vi "Calibration Mode.vi"(8 "error in (no error)":errorcluster, 10 "Enable":bool, 11 "ENET in":refnum<class "ENET_BS120x.lvclass">) -> (0 "error out":errorcluster, 3 "ENET out":refnum<class "ENET_BS120x.lvclass">)   [LabVIEW 2021, in "BS120x Driver.lvlib" / "ENET_BS120x.lvclass"]
doc: "Calibration mode disables the current calibration, removes all scaling, and returns bit counts."
uses:
  ENET_BS120x.lvclass
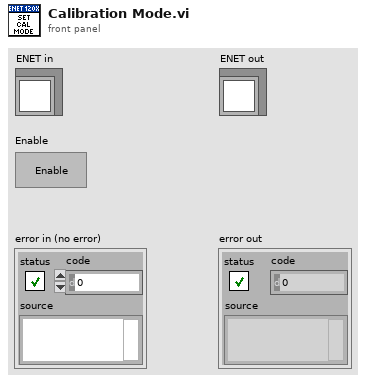
[diagram p1: front panel]
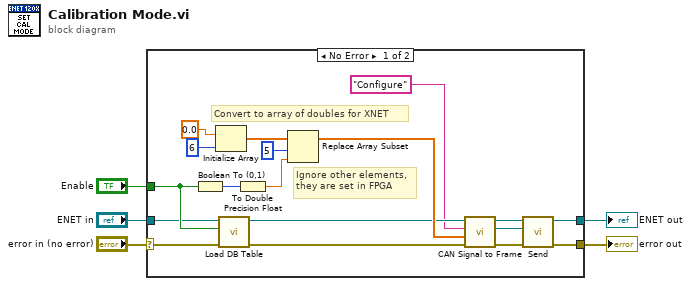
[diagram p0: block diagram]
diagram:
  n1 = case shown="No Error" "error in (no error)" {
    selector: "error in (no error)" -> [w23 w25]
    tunnel: [w8 w25] -> w4
    tunnel: [w9 w24] -> w2
    tunnel: "ENET in" -> [w15 w24]
    tunnel: "Enable" -> [w16 _]
    frame No Error {
      # "Ignore other elements,\nthey are set in FPGA"
      # "Convert to array of doubles for XNET"
      n2 = Boolean To (0,1)(Boolean=w16) -> (0, 1=w17:i16)
      n3 = Initialize Array(0.0 ("element"), 6 ("dimension size")) -> (w21:dbl[])
      n4 = call-dynamic "Load DB Table.vi"("error in (no error)"=w23, "Calibration Mode"=w16, "ENET in"=w15) -> ("error out"=w6:errorcluster, "ENET out"=w13:refnum<class "ENET_BS120x.lvclass">)  [unwired: 7 in]
      n5 = To Double Precision Float(number=w17) -> (double precision float=w22:dbl)
      n6 = Replace Array Subset(array=w21, new element=w22, index=5) -> (w14:dbl[])
      n7 = call "CAN Signal to Frame.vi"("error in (no error)"=w6, "Data Array"=w14, "Frame"="Configure", "ENET in"=w13) -> ("error out"=w7:errorcluster, "Data"=w10:refnum<class "Data.lvclass">, "ENET out"=w11:refnum<class "ENET_BS120x.lvclass">)  [unwired: 5 in]
      n8 = call "Send.vi"("error in (no error)"=w7, "Data"=w10, "ENET in"=w11) -> ("error out"=w8:errorcluster, "ENET out"=w9:refnum<class "ENET_BS120x.lvclass">)  [unwired: 7 in]
    }
    frame Error {
    }
  }
  "error out" <- w4
  "ENET out" <- w2
